vi "GetMTRTYield.vi"(10 "RCNO":string="A150100736") -> (2 "Array":dbl[](array[numeric]))   [LabVIEW 2012]
uses:
  <vilib>/addons/database/Auxilliary.llb/DB Tools Cursor Type.ctl
  <vilib>/addons/database/Connection.llb/DB Tools Open Connec (Path).vi
  <vilib>/addons/database/Connection.llb/Conn Execute.vi
  <vilib>/addons/database/Recordset.llb/Rec Fetch Integer Data (R).vi
  <vilib>/addons/database/Recordset.llb/Rec Destroy - Connection.vi
  <vilib>/addons/database/NI_Database_API.lvlib
panel:
  out "concatenated string":string
  out "error out":errorcluster
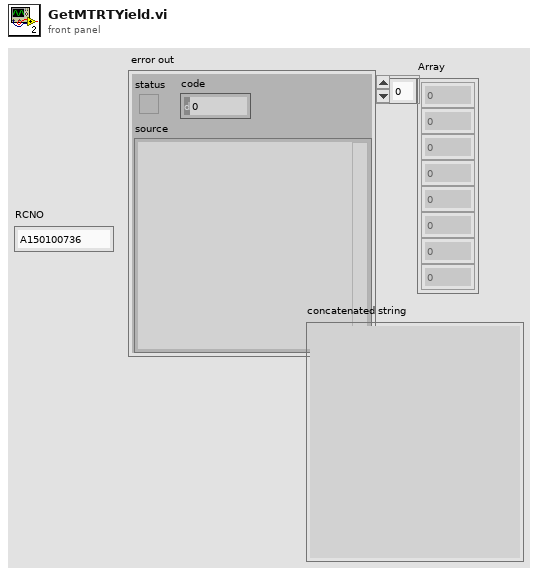
[diagram p1: front panel]
types:
  T1 = typedef "NI_Database_API.lvlib/Conn ObjectReference.ctl" = refnum<k1>
  T2 = typedef "NI_Database_API.lvlib/DB Tools Cursor Type.ctl" = enum16{"forward-only", "keyset", "dynamic", "static"}
  T3 = typedef "NI_Database_API.lvlib/Rec ObjectReference.ctl" = refnum<k1>
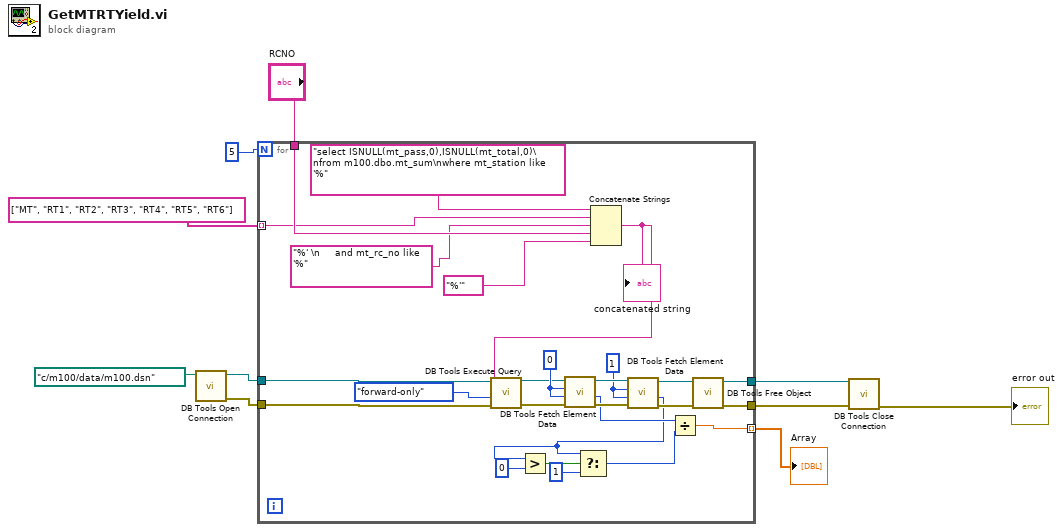
[diagram p0: block diagram]
diagram:
  n1 = call-poly <vilib>:"DB Tools Open Connection.vi"("connection information"=path "c:/m100/data/m100.dsn") -> ("error out"=w8:errorcluster, "connection reference"=w9:T1)  [unwired: 7 in]
  n2 = for {
    N: 5 -> [_]
    tunnel: w9 -> [w36]
    tunnel: w8 -> [w35]
    tunnel: "RCNO" -> [w22]
    tunnel: string[] ["MT", "RT1", "RT2", "RT3", "RT4", "RT5", "RT6"] -> [w17] mode=indexing
    tunnel: [w21] -> w3
    tunnel: [w20] -> w2
    tunnel: [w19] -> w1 mode=indexing
    w32 = 1
    w28 = 0
    n3 = Concatenate Strings("select ISNULL(mt_pass,0),ISNULL(mt_total,0)\nfrom m100.dbo.mt_sum\nwhere mt_station like '%", w17, "%' \n     and mt_rc_no like '%" ("string"), w22, "%'" ("string")) -> (w29:string)
    "concatenated string" <- w29
    n4 = call-poly <vilib>:"DB Tools Execute Query.vi"("error in (no error)"=w35, "cursor type"=DB_Tools_Cursor_Type."forward-only", "SQL query"=w29, "connection reference"=w36) -> ("error out"=w26:errorcluster, "recordset reference"=w27:T3)  [unwired: 4 in]
    n5 = call-poly <vilib>:"DB Tools Fetch Element Data.vi"("error in (no error)"=w26, "type"=w28, "column index"=w28, "recordset reference"=w27) -> ("error out"=w34:errorcluster, "data"=w24:i32, "recordset reference out"=w33:T3)  [unwired: 3 in]
    n6 = call-poly <vilib>:"DB Tools Fetch Element Data.vi"("error in (no error)"=w34, "type"=w32, "column index"=w32, "recordset reference"=w33) -> ("error out"=w30:errorcluster, "data"=w14:i32, "recordset reference out"=w31:T3)  [unwired: 3 in]
    n7 = Greater?(x=w14, y=0) -> (0:w15:bool)
    n8 = Select(t=w14, s=w15, f=1) -> (s? t:f=w11:i32)
    n9 = Divide(x=w24, y=w11) -> (x/y=w19:dbl)
    n10 = call-poly <vilib>:"DB Tools Free Object.vi"("error in (no error)"=w30, "recordset reference"=w31) -> ("error out"=w20:errorcluster, "connection reference"=w21:T1)  [unwired: 8 in]
  }
  "Array" <- w1
  n11 = call <vilib>:"DB Tools Close Connection.vi"("error in (no error)"=w2, "connection reference"=w3) -> ("error out"=→"error out":errorcluster)  [unwired: 5 in]
